vi "As Minimal Cluster.vi"(8 "error in (no error)":errorcluster, 11 "Parameter to Hardware Map in":refnum<class "Parameter to Hardware Map.lvclass">) -> (0 "error out":errorcluster, 2 "Minimal Parameter to Hardware Map out":T1, 3 "Parameter to Hardware Map out":refnum<class "Parameter to Hardware Map.lvclass">)   [LabVIEW 2020, in "Parameter to Hardware Map.lvclass"]
doc: "Returns a minimal representation of the entire map using only serializable data types (mostly strings, arrays, and clusters)"
uses:
  Parameter to Hardware Map.lvclass
  Controller/Minimal Controller Cluster.ctl
  Controller/Generic Plugin.lvclass
  Minimal Map.ctl
  Minimal Pair Cluster.ctl
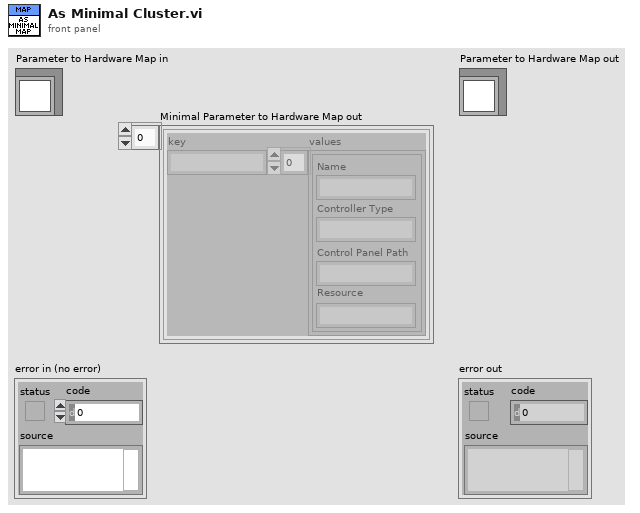
[diagram p1: front panel]
types:
  T1 = typedef "Parameter to Hardware Map.lvclass/Minimal Map.ctl" = T2[]
  T2 = typedef "Parameter to Hardware Map.lvclass/Minimal Pair Cluster.ctl" = cluster{"key":string, "values":T3[]}
  T3 = typedef "Generic Plugin.lvclass/Minimal Controller Cluster.ctl" = cluster{"Name":string, "Controller Type":string, "Control Panel Path":string, "Resource":string}
  T4 = typedef "Parameter to Hardware Map.lvclass/Pair.ctl" = cluster{"key":string, "values":refnum<class "Generic Plugin.lvclass">[]}
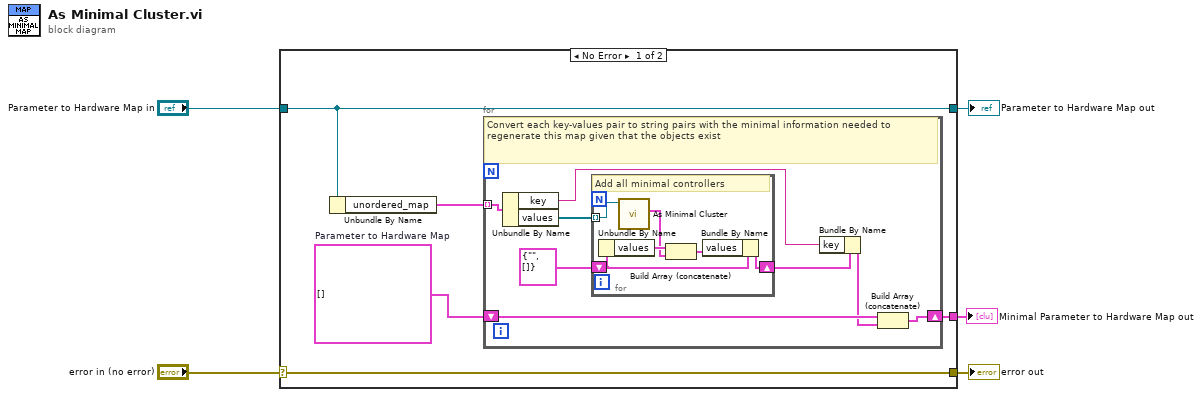
[diagram p0: block diagram]
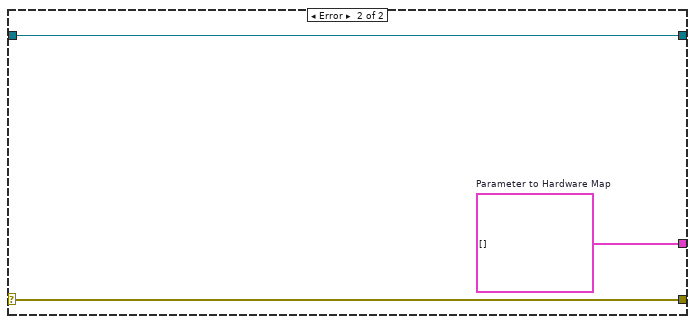
[diagram p2: hidden frame]
diagram:
  n1 = case shown="No Error" "error in (no error)" {
    selector: "error in (no error)" -> [w10 w27]
    tunnel: [w10 w27] -> w4
    tunnel: [w9 w26] -> w2
    tunnel: "Parameter to Hardware Map in" -> [w9 w26]
    tunnel: [w6 w25] -> w1
    frame No Error {
      w7 = T1 []  # Parameter to Hardware Map
      n2 = Unbundle By Name(w9) -> ("unordered_map"=w8:T4[])
      n3 = for {
        tunnel: w8 -> [w18] mode=indexing
        shift-right: [w13] -> w6
        shift-left: w7 -> [w14]
        # "Convert each key-values pair to string pairs with the minimal information needed to regenerate this map given that the objects exist"
        n4 = Unbundle By Name(w18) -> ("key"=w11:string, "values"=w17:refnum<class "Generic Plugin.lvclass">[])
        n5 = for {
          tunnel: w17 -> [w24] mode=indexing
          shift-right: [w23] -> w15
          shift-left: T2 {"key"="", "values"=[]} ("Pair") -> [w22]
          # "Add all minimal controllers"
          n6 = Unbundle By Name(w22) -> ("values"=w21:T3[])
          n7 = call-dynamic "As Minimal Cluster.vi"("Generic Controller in"=w24) -> ("Minimal Cluster out"=w19:T3)  [unwired: 8 in, 2 out]
          n8 = Build Array (concatenate)(w21, w19) -> (w20:T3[])
          n9 = Bundle By Name(cluster=w22, "values"=w20) -> (w23:T2)
        }
        n10 = Bundle By Name(cluster=w15, "key"=w11) -> (w12:T2)
        n11 = Build Array (concatenate)(w14, w12) -> (w13:T1)
      }
    }
    frame Error {
      w25 = T1 []  # Parameter to Hardware Map
    }
  }
  "error out" <- w4
  "Parameter to Hardware Map out" <- w2
  "Minimal Parameter to Hardware Map out" <- w1
